vi "Логический блок.vi"(1 "c":T1, 2 "b":bool, 3 "a":bool) -> (0 "r":bool)   [LabVIEW 2013]
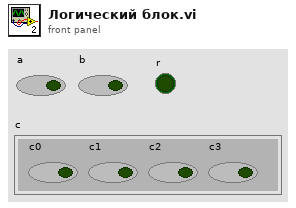
[diagram p1: front panel]
types:
  T1 = cluster{"c0":bool, "c1":bool, "c2":bool, "c3":bool}
  T2 = cluster{bool, bool, bool, "a":bool, bool, "b":bool, bool, bool, bool, bool, bool, bool, bool, bool, bool, bool}
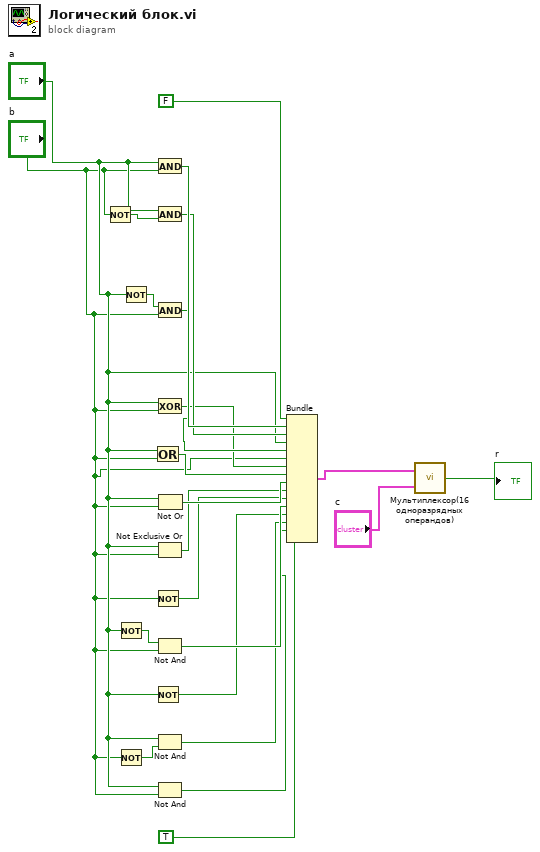
[diagram p0: block diagram]
diagram:
  n1 = Not(x="b") -> (.not. x?=w23:bool)
  n2 = Not(x="a") -> (.not. x?=w21:bool)
  n3 = Not(x="b") -> (.not. x?=w20:bool)
  n4 = Not(x="a") -> (.not. x?=w22:bool)
  n5 = Or(x="a", y="b") -> (x .or. y?=w14:bool)
  n6 = Not(x="b") -> (.not. x?=w11:bool)
  n7 = Not(x="a") -> (.not. x?=w9:bool)
  n8 = And(x="a", y="b") -> (x .and. y?=w18:bool)
  n9 = And(x="a", y=w23) -> (x .and. y?=w17:bool)
  n10 = And(x=w22, y="b") -> (x .and. y?=w16:bool)
  n11 = Exclusive Or(1:"b", 2:"a") -> (0:w15:bool)
  n12 = Not Or(1:"b", 2:"a") -> (0:w13:bool)
  n13 = Not Exclusive Or(1:"b", 2:"a") -> (0:w12:bool)
  n14 = Not And(1:"b", 2:w21) -> (0:w10:bool)
  n15 = Not And(1:w20, 2:"a") -> (0:w8:bool)
  n16 = Not And(1:"b", 2:"a") -> (0:w7:bool)
  n17 = Bundle(FALSE, w18, w17, "a"="a", w16, "b"="b", w15, w14, w13, w12, w11, w10, w9, w8, w7, TRUE) -> (w3:T2)  [unwired: 1 in]
  n18 = call "Мультиплексор(16 одноразрядных операндов).vi"("c"="c", "in"=w3) -> ("r"=→"r":bool)
